vi "PlayerName.vi"(8 "error in (no error)":errorcluster, 9 "VI Refnum":refnum<vi>, 10 "PlayerName":string, 11 "simonMessages in":refnum<class "simonMessages.lvclass">) -> (0 "error out":errorcluster, 3 "simonMessages out":refnum<class "simonMessages.lvclass">)   [LabVIEW 2019, in "simonMessages.lvclass"]
uses:
  simonMessages.lvclass
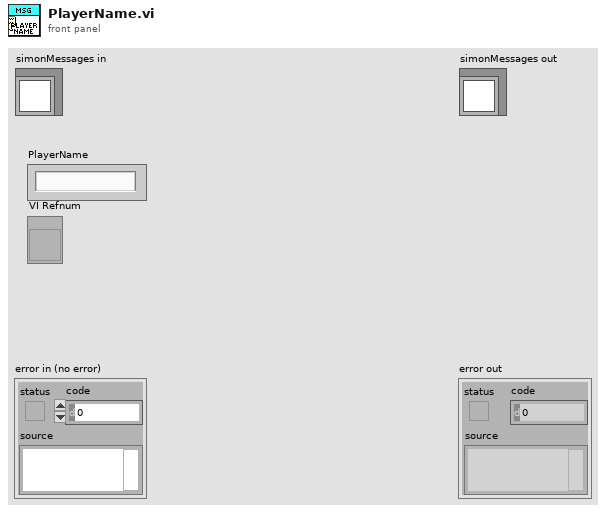
[diagram p1: front panel]
types:
  T1 = cluster{"Text":string, "Size":u8, "Justification":enum16{"Left", "Center", "Right"}, "Display Type":string}
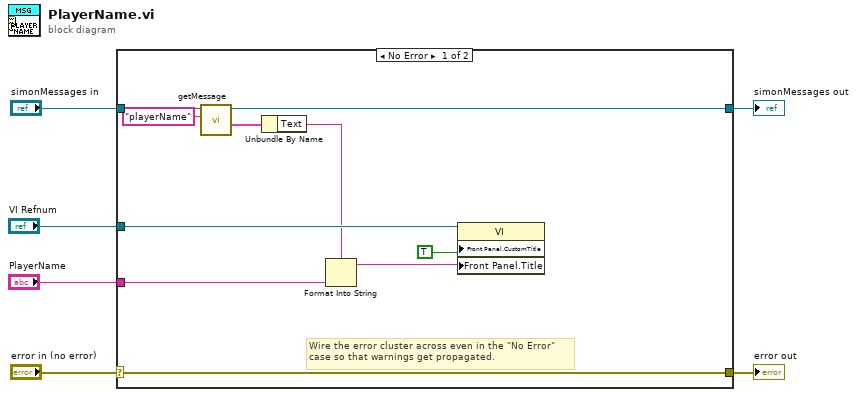
[diagram p0: block diagram]
diagram:
  n1 = case shown="No Error" "error in (no error)" {
    selector: "error in (no error)" -> [w15 w18]
    tunnel: [w15 w18] -> w5
    tunnel: [w14 w17] -> w3
    tunnel: "simonMessages in" -> [w16 w17]
    tunnel: "VI Refnum" -> [w11 _]
    tunnel: "PlayerName" -> [w9 _]
    frame No Error {
      # "Wire the error cluster across even in the \"No Error\"\ncase so that warnings get propagated."
      n2 = call "getMessage.vi"("key"="playerName", "simonMessages in"=w16) -> ("Message Cluster"=w10:T1, "simonMessages out"=w14:refnum<class "simonMessages.lvclass">)  [unwired: 7 in, 1 out]
      n3 = Unbundle By Name(w10) -> ("Text"=w7:string)
      n4 = Format Into String(format string=w7, w9) -> (resulting string=w8:string)  [unwired: 2 in, 1 out]
      n5 = property class="VI"(reference=w11, "Front Panel.CustomTitle"=TRUE ("Front Panel Window:Custom Title"), "Front Panel.Title"=w8) -> ()  [unwired: 1 in, 2 out]
    }
    frame Error {
    }
  }
  "error out" <- w5
  "simonMessages out" <- w3
